vi "读取VISA resource name.vi"(8 "error in (no error)":errorcluster caption="错误输入（无错误）", 11 "DMM输入":refnum<class "DMM.lvclass">) -> (0 "error out":errorcluster caption="错误输出", 2 "VISA resource name":refnum<visa-resource-name>, 3 "DMM输出":refnum<class "DMM.lvclass">)   [LabVIEW 2020, in "DMM.lvlib" / "DMM.lvclass"]
uses:
  DMM.lvclass
  DMM.lvclass/DMM.ctl
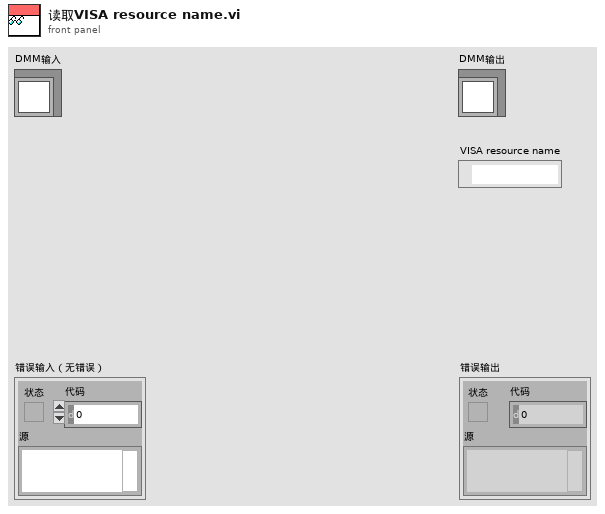
[diagram p1: front panel]
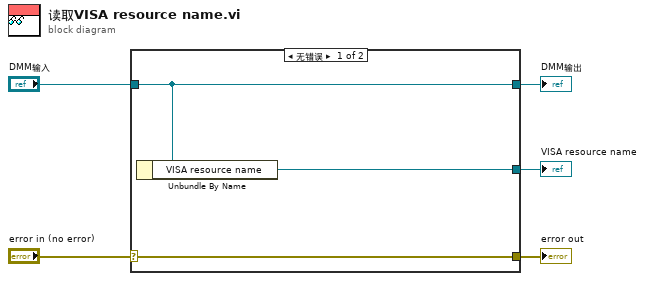
[diagram p0: block diagram]
diagram:
  n1 = case shown="无错误" "error in (no error)" {
    selector: "error in (no error)" -> [w8 w9]
    tunnel: [w8 w9] -> w4
    tunnel: [w7 w10] -> w2
    tunnel: "DMM输入" -> [w7 w10]
    tunnel: [w6 _] -> w1
    frame No Error {
      n2 = Unbundle By Name(w7) -> ("VISA resource name"=w6:refnum<visa-resource-name>)
    }
    frame Error {
    }
  }
  "error out" <- w4
  "DMM输出" <- w2
  "VISA resource name" <- w1
